vi "NRZ Encoder (SubVI).vi"(11 "Input Bit":i32) -> (3 "NRZ Output":dbl)   [LabVIEW 2026]
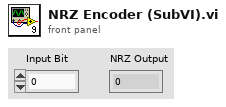
[diagram p1: front panel]
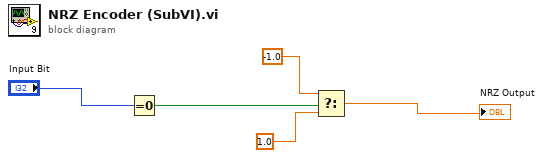
[diagram p0: block diagram]
diagram:
  n1 = Equal To 0?(x="Input Bit") -> (x = 0?=w4:bool)
  n2 = Select(t=-1.0, s=w4, f=1.0) -> (s? t:f=→"NRZ Output":dbl)
